vi "Ballard 429 - Parse Message.vi"(8 "Error (in)":errorcluster, 9 "Inline Status Channels Refs":T1[](array[typedef]) format="%.0x", 10 "Record []":T13[](array[typedef]) {"type" format="%04x"; "timestamp" format="%08x"; "msgact" format="%04x"; "data" format="%08x"; "timestamph" format="%08x"}, 11 "Channel Data [] In":T2[](array[typedef])=[{"Labels Settings"=[{"Name"="", "xmlName"="", "Label"=0, "transferPeriod"=0, "SDI_Enabled"=FALSE, "SDI"=0, "Word"={"Param Setting"={"Start Bit"=[], "Num Bits"=[], "Signed?"=[], "ScaleFac"=[], "ScaleOffset"=[], "Block Data Refs"=[], "Encoding"=[], "Values Array"=[], "Item Refs"=[]}}, "TransferType"=enum."ScheduledLabel", "has timestamp?"=FALSE, "Label Disable/Trigger Channel Reference"=0, "Message Handle"=0, "Initialized?"=FALSE, "Word Initial Raw Value"=0, "Label Timestamp Channel Data Reference"=0}], "channel handle"=0, "channel #"=0}] {"Labels Settings"."Label Timestamp Channel Data Reference" format="%.0x"; "Labels Settings"."Label Disable/Trigger Channel Reference" format="%.0x"; "Labels Settings"."Word"."Param Setting"."Item Refs" format="%.0x"; "Labels Settings"."Word"."Param Setting"."Num Bits" min=1 max=32; "Labels Settings"."Word"."Param Setting"."Start Bit" min=8 max=31; "Labels Settings"."Label" format="%.0o"}) -> (0 "Error (out)":errorcluster)   [LabVIEW 2020, in "Ballard Arinc-429 Engine.lvlib"]
uses:
  Ballard Arinc-429 Engine.lvlib
  <instrlib>/BTICardLib/Public/Controls/429 Record.ctl
  Shared/Controls and Global/RT HW Channel.ctl
  Shared/Controls and Global/RT Label Settings.ctl
  Shared/Controls and Global/Label.ctl
  Shared/Controls and Global/transferPeriod.ctl
  Shared/Controls and Global/RT Word Settings.ctl
  Shared/Controls and Global/RT Param Setting.ctl
  Shared/Controls and Global/Start Bit.ctl
  Shared/Controls and Global/Number of Bits.ctl
  <vilib>/NI VeriStand/Custom Device API/Block Data Reference.ctl
  <vilib>/NI VeriStand/Custom Device API/Data Reference.ctl
  <vilib>/NI VeriStand/Custom Device API/Custom Device Item Ref.ctl
  Shared/Controls and Global/TransferType.ctl
  Extract BCD Parameter.vi
  <vilib>/NI VeriStand/Custom Device API/Global Data Refs.vi
  <instrlib>/BTI429Lib/BTI429LV.lvlib
  Shared/Ballard Arinc-429 Shared.lvlib
  <vilib>/NI VeriStand/Custom Device API/Custom Device API.lvlib
  <vilib>/NI VeriStand/Custom Device Tools/Custom Device Utility Library/Custom Device Utility Library.lvlib
  <instrlib>/BTI429Lib/Private/Utility/Get Fld SDI.vi
  <instrlib>/BTICardLib/BTICardLV.lvlib
panel:
  out "Label # 2":i32
  out "Waveform Chart 2":i32(graph)
  out "source/destination identifiers (SDI) out 2":u8 format="%02b"
  out "Physical Channel # 2":i32
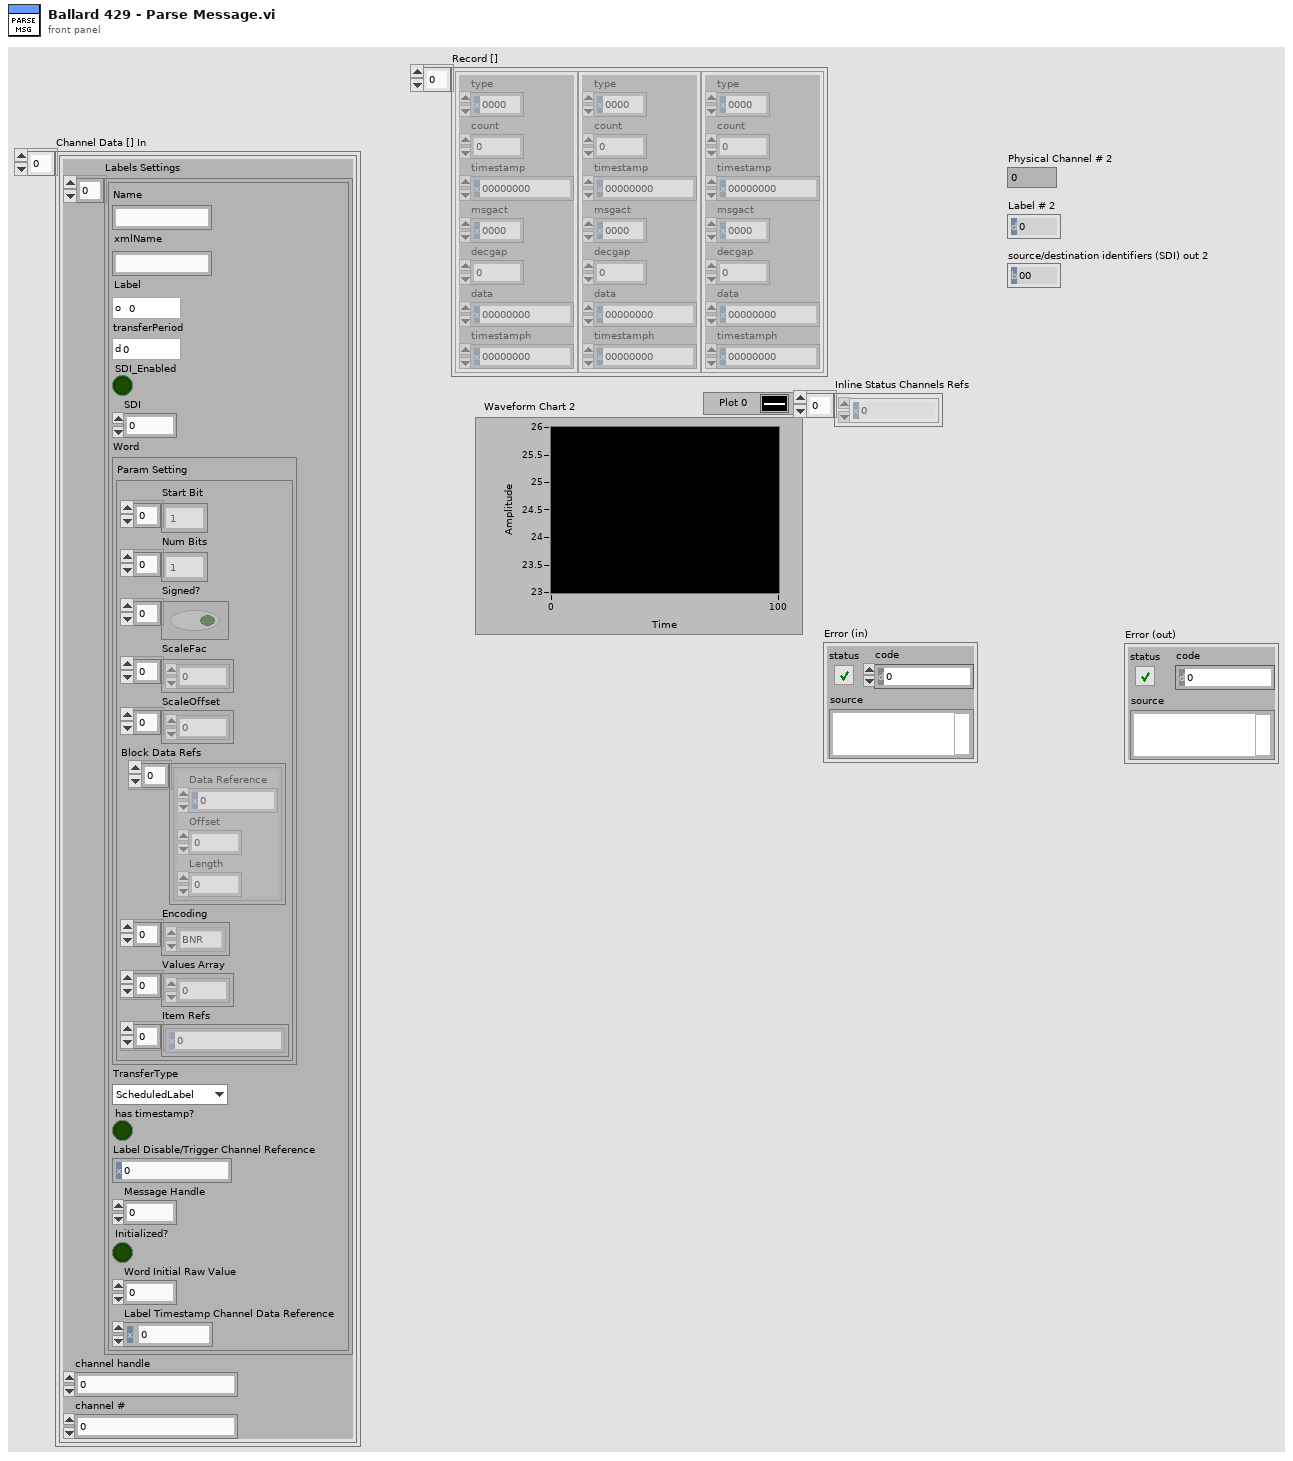
[diagram p1: front panel]
types:
  T1 = typedef "Custom Device API.lvlib/Data Reference.ctl" = i32
  T2 = typedef "Ballard Arinc-429 Shared.lvlib/RT HW Channel.ctl" = cluster{"Labels Settings":T3[], "channel handle":u64, "channel #":u16}
  T3 = typedef "Ballard Arinc-429 Shared.lvlib/RT Label Settings.ctl" = cluster{"Name":string, "xmlName":string, "Label":T4, "transferPeriod":T5, "SDI_Enabled":bool, "SDI":u8, "Word":T6, "TransferType":T12, "has timestamp?":bool, "Label Disable/Trigger Channel Reference":T11, "Message Handle":u64, "Initialized?":bool, "Word Initial Raw Value":u32, "Label Timestamp Channel Data Reference":T1}
  T4 = typedef "Ballard Arinc-429 Shared.lvlib/Label.ctl" = u8
  T5 = typedef "Ballard Arinc-429 Shared.lvlib/transferPeriod.ctl" = u32
  T6 = typedef "Ballard Arinc-429 Shared.lvlib/RT Word Settings.ctl" = cluster{"Param Setting":T7}
  T7 = typedef "Ballard Arinc-429 Shared.lvlib/RT Param Setting.ctl" = cluster{"Start Bit":T8[], "Num Bits":T9[], "Signed?":bool[], "ScaleFac":dbl[], "ScaleOffset":dbl[], "Block Data Refs":T10[], "Encoding":enum16{"BNR", "BCD", "Discrete"}[], "Values Array":dbl[], "Item Refs":T11[]}
  T8 = typedef "Ballard Arinc-429 Shared.lvlib/Start Bit.ctl" = i32
  T9 = typedef "Ballard Arinc-429 Shared.lvlib/Number of Bits.ctl" = i32
  T10 = typedef "Custom Device API.lvlib/Block Data Reference.ctl" = cluster{"Data Reference":T1, "Offset":u64, "Length":u64}
  T11 = typedef "Custom Device API.lvlib/Custom Device Item Ref.ctl" = u64
  T12 = typedef "Ballard Arinc-429 Shared.lvlib/TransferType.ctl" = enum16{"ScheduledLabel", "Acyclic", "Block", "Strobe"}
  T13 = typedef "BTICardLV.lvlib/429 Record.ctl" = cluster{"type":u16, "count":u16, "timestamp":u32, "msgact":u16, "decgap":u16, "data":u32, "timestamph":u32}
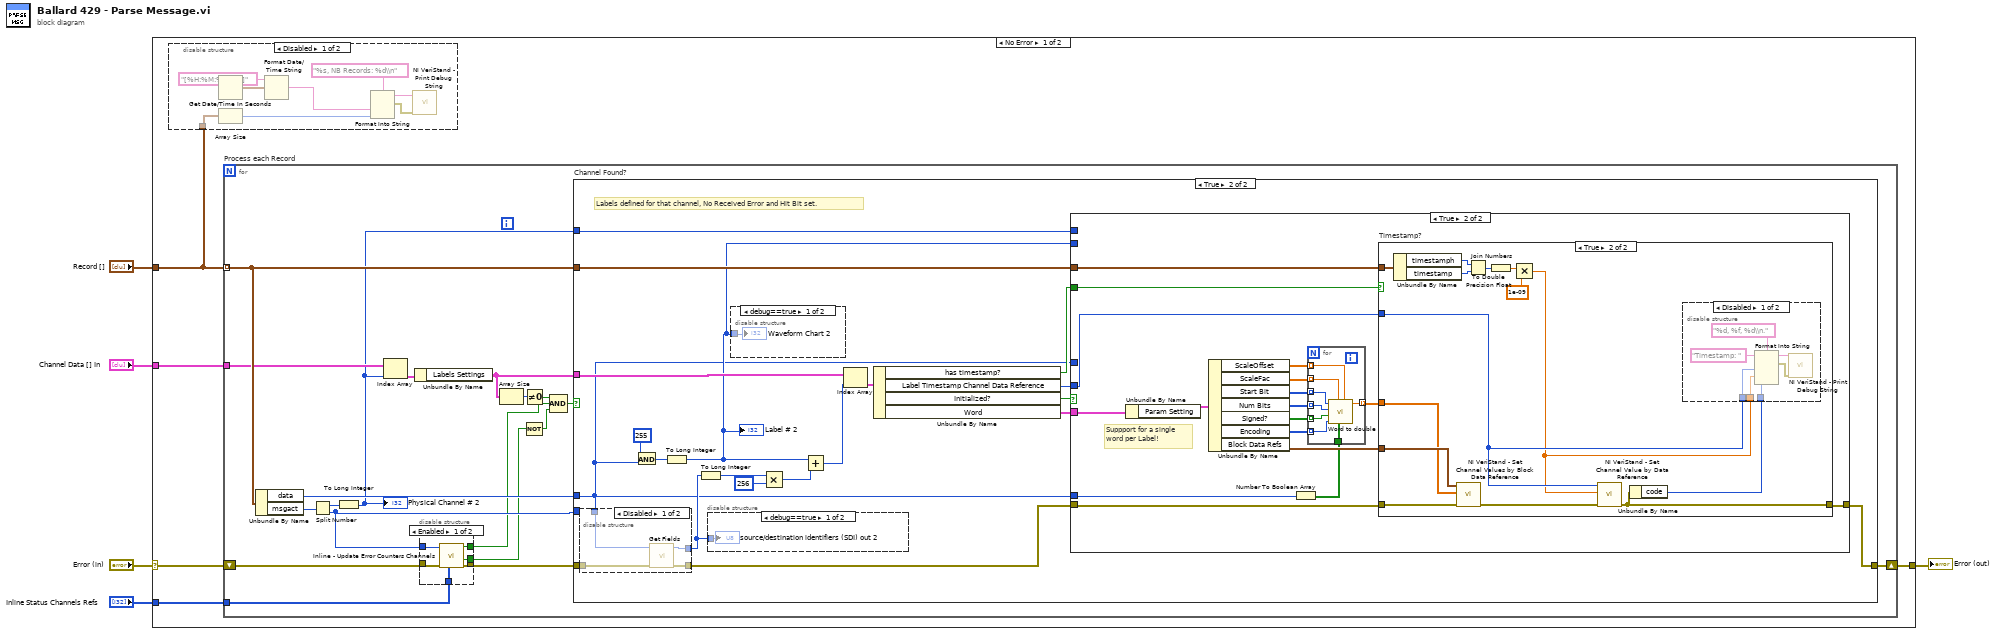
[diagram p0: block diagram]
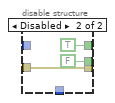
[diagram p3: hidden frame]
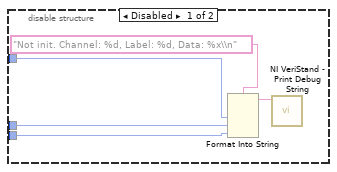
[diagram p6: hidden frame]
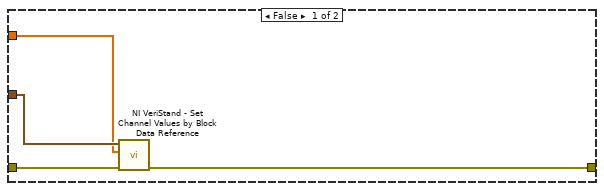
[diagram p7: hidden frame]
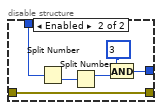
[diagram p11: hidden frame]
diagram:
  n1 = case shown="No Error" "Error (in)" {
    selector: "Error (in)" -> [w8 w139]
    tunnel: "Record []" -> [w7 _]
    tunnel: [w10 w139] -> w4
    tunnel: "Channel Data [] In" -> [w9 _]
    tunnel: "Inline Status Channels Refs" -> [w6 _]
    frame No Error {
      n2 = disable-structure shown="Disabled" {
        disable-tunnel: w7 -> [w18 _]
        frame Disabled {
          n3 = Get Date/Time In Seconds() -> (seconds since 1Jan1904=w17:timestamp)
          n4 = Array Size(array=w18) -> (size(s)=w15:i32)
          n5 = Format Date/Time String(time format string (%c)="[%H:%M:%S%3u]", seconds (now)=w17) -> (date/time string=w16:string)  [unwired: 1 in]
          n6 = Format Into String(format string="%s, NB Records: %d\\n", w16, w15) -> (resulting string=w11:string, error out=w12:errorcluster)  [unwired: 2 in]
          n7 = call <vilib>:"NI VeriStand - Print Debug String.vi"("error in (no error)"=w12, "Message"=w11) -> ()  [unwired: 9 in, 1 out]
        }
        frame Enabled {
        }
      }
      n8 = for "Process each Record" {
        tunnel: w7 -> [w37] mode=indexing
        shift-right: [w23] -> w10
        shift-left: w8 -> [w35]
        tunnel: w9 -> [w36]
        tunnel: w6 -> [w27]
        n9 = Unbundle By Name(w37) -> ("data"=w34:u32, "msgact"=w33:u16)
        n10 = Split Number(x=w33) -> (hi(x)=w31:u8, lo(x)=w26:u8)
        n11 = To Long Integer(number=w31) -> (32bit integer=w28:i32)
        "Physical Channel # 2" <- w28
        n12 = Index Array(array=w36, index=w28) -> (element=w29:T2)
        n13 = Unbundle By Name(w29) -> ("Labels Settings"=w30:T3[])
        n14 = disable-structure shown="Enabled" {
          disable-tunnel: w35 -> [w43 w46]
          disable-tunnel: w27 -> [w42 _]
          disable-tunnel: w26 -> [w41 _]
          disable-tunnel: [w40 w46] -> w25
          disable-tunnel: [w39 FALSE ("Bit Error")] -> w24
          disable-tunnel: [w38 TRUE ("Hit")] -> w20
          frame Enabled {
            n15 = call "Inline - Update Error Counters Channels.vi"("Inline Status Channels Refs"=w42, "error in (no error)"=w43, "msgact"=w41) -> ("error IO"=w40:errorcluster, "Bit Error"=w39:bool, "Hit"=w38:bool)  [unwired: 6 in]
          }
          frame Disabled {
          }
        }
        n16 = Array Size(array=w30) -> (size(s)=w32:i32)
        n17 = Not(x=w24) -> (.not. x?=w19:bool)
        n18 = Not Equal To 0?(x=w32) -> (x != 0?=w22:bool)
        n19 = Compound Arithmetic op=AND(w22, w20, w19) -> (w21:bool)
        n20 = case "Channel Found?" shown="True" w21 {
          tunnel: w25 -> [w47 w65]
          tunnel: [w47 w54] -> w23
          tunnel: w34 -> [_ w48]
          tunnel: w37 -> [_ w67]
          tunnel: w30 -> [_ w59]
          tunnel: w28 -> [_ w49]
          tunnel: w26 -> [_ _]
          frame False {
            # "No Labels configured for that channel or no HIT or Error."
          }
          frame True {
            # "Labels defined for that channel, No Received Error and Hit Bit set."
            n21 = disable-structure shown="Disabled" {
              disable-tunnel: w48 -> [w132 w137]
              disable-tunnel: w65 -> [w131 w138]
              disable-tunnel: [w130 w138] -> w55
              disable-tunnel: [w129 w135] -> w64
              frame Disabled {
                n22 = call-poly <instrlib>:"Get Fields.vi"("error in (no error)"=w131, "message"=w132) -> ("error out"=w130:errorcluster, "source/destination identifiers (SDI) out"=w129:u16)  [unwired: 8 in]
              }
              frame Enabled {
                n23 = Split Number(x=w137) -> (lo(x)=w136:u16)  [unwired: 1 out]
                n24 = Split Number(x=w136) -> (hi(x)=w134:u8)  [unwired: 1 out]
                n25 = And(x=u8 3, y=w134) -> (x .and. y?=w135:u8)
              }
            }
            n26 = And(x=u32 255 ("y"), y=w48) -> (x .and. y?=w66:u32)
            n27 = To Long Integer(number=w66) -> (32bit integer=w50:i32)
            "Label # 2" <- w50
            n28 = To Long Integer(number=w64) -> (32bit integer=w63:i32)
            n29 = disable-structure shown="debug==true" {
              disable-tunnel: w64 -> [w127 _]
              frame condition #0 {
                "source/destination identifiers (SDI) out 2" <- w127
              }
              frame condition #1 (active) {
              }
            }
            n30 = disable-structure shown="debug==true" {
              disable-tunnel: w50 -> [w128 _]
              frame condition #0 {
                "Waveform Chart 2" <- w128
              }
              frame condition #1 (active) {
              }
            }
            n31 = Multiply(x=w63, y=256) -> (x*y=w62:i32)
            n32 = Add(x=w50, y=w62) -> (x+y=w58:i32)
            n33 = Index Array(array=w59, index=w58) -> (element=w56:T3)
            n34 = Unbundle By Name(w56) -> ("has timestamp?"=w52:bool, "Label Timestamp Channel Data Reference"=w51:T1, "Initialized?"=w53:bool, "Word"=w57:T6)
            n35 = case shown="True" w53 {
              tunnel: w57 -> [_ w91]
              tunnel: w67 -> [_ w93]
              tunnel: w48 -> [_ w92]
              tunnel: w55 -> [w71 w87]
              tunnel: [w71 w88] -> w54
              tunnel: w52 -> [_ w90]
              tunnel: w51 -> [_ w89]
              tunnel: w50 -> [w69 _]
              tunnel: w49 -> [w70 _]
              tunnel: w48 -> [w68 _]
              frame False {
                # "This case will be called if users has Labels present on the channel but didn't list them in XML file with \"monitor=false\" in the list.\nRecords returned by Read function will have this labels (not filtered by HW)."
                n36 = disable-structure shown="Enabled" {
                  disable-tunnel: w70 -> [w75 _]
                  disable-tunnel: w69 -> [w74 _]
                  disable-tunnel: w68 -> [w72 _]
                  frame Disabled {
                    n37 = Format Into String(format string="Not init. Channel: %d, Label: %d, Data: %x\\n" ("initial string"), w75, w74, w72) -> (resulting string=w73:string)  [unwired: 2 in, 1 out]
                    n38 = call <vilib>:"NI VeriStand - Print Debug String.vi"("Message"=w73) -> ()  [unwired: 10 in, 1 out]
                  }
                  frame Enabled {
                  }
                }
              }
              frame True {
                # "Suppport for a single\nword per Label!"
                n39 = Unbundle By Name(w91) -> ("Param Setting"=w86:T7)
                n40 = Unbundle By Name(w86) -> ("ScaleOffset"=w80:dbl[], "ScaleFac"=w85:dbl[], "Start Bit"=w84:T8[], "Num Bits"=w83:T9[], "Signed?"=w82:bool[], "Encoding"=w79:enum16{"BNR", "BCD", "Discrete"}[], "Block Data Refs"=w78:T10[])
                n41 = Number To Boolean Array(number=w92) -> (Boolean array=w77:bool[])
                n42 = for {
                  tunnel: [w126] -> w81 mode=indexing
                  tunnel: w80 -> [w125] mode=indexing
                  tunnel: w85 -> [w124] mode=indexing
                  tunnel: w84 -> [w123] mode=indexing
                  tunnel: w83 -> [w122] mode=indexing
                  tunnel: w82 -> [w121] mode=indexing
                  tunnel: w79 -> [w120] mode=indexing
                  tunnel: w77 -> [w119]
                  n43 = call "Word to double.vi"("ScaleOffset (0)"=w125, "Word"=w119, "ScaleFac (1)"=w124, "Encoding"=w120, "Signed? (F)"=w121, "Number of Bits"=w122, "Start Bit"=w123) -> ("Double"=w126:dbl)  [unwired: 4 in]
                }
                n44 = case "Timestamp?" shown="True" w90 {
                  tunnel: w81 -> [w94 w102]
                  tunnel: w93 -> [_ w106]
                  tunnel: w78 -> [w95 w103]
                  tunnel: w87 -> [w97 w105]
                  tunnel: [w96 w99] -> w88
                  tunnel: w89 -> [_ w101]
                  frame False {
                    n45 = call <vilib>:"NI VeriStand - Set Channel Values by Block Data Reference.vi"("error in (no error)"=w97, "Values Array in"=w94, "Block Data Ref"=w95) -> ("error out"=w96:errorcluster)  [unwired: 6 in, 2 out]
                  }
                  frame True {
                    n46 = Unbundle By Name(w106) -> ("timestamph"=w111:u32, "timestamp"=w110:u32)
                    n47 = call <vilib>:"NI VeriStand - Set Channel Values by Block Data Reference.vi"("error in (no error)"=w105, "Values Array in"=w102, "Block Data Ref"=w103) -> ("error out"=w104:errorcluster)  [unwired: 6 in, 2 out]
                    n48 = Join Numbers(hi=w111, lo=w110) -> ((hi.lo)=w109:u64)
                    n49 = To Double Precision Float(number=w109) -> (double precision float=w108:dbl)
                    n50 = Multiply(x=w108, y=1e-09) -> (x*y=w100:dbl)
                    n51 = call <vilib>:"NI VeriStand - Set Channel Value by Data Reference.vi"("error in (no error)"=w104, "Value"=w100, "Data Reference in"=w101) -> ("error out"=w99:errorcluster)  [unwired: 8 in]
                    n52 = Unbundle By Name(w99) -> ("code"=w98:i32)
                    n53 = disable-structure shown="Disabled" {
                      disable-tunnel: w101 -> [w118 _]
                      disable-tunnel: w100 -> [w117 _]
                      disable-tunnel: w98 -> [w116 _]
                      frame Disabled {
                        n54 = Format Into String(format string="%d, %f, %d\\n.", initial string="Timestamp: ", w118, w117, w116) -> (resulting string=w114:string, error out=w115:errorcluster)  [unwired: 1 in]
                        n55 = call <vilib>:"NI VeriStand - Print Debug String.vi"("error in (no error)"=w115, "Message"=w114) -> ()  [unwired: 9 in, 1 out]
                      }
                      frame Enabled {
                      }
                    }
                  }
                }
              }
            }
          }
        }
      }
    }
    frame Error {
    }
  }
  "Error (out)" <- w4
